vi "top level batch unzip VI.vi"() -> ()   [LabVIEW 2010]
uses:
  <vilib>/zip/NI_Unzip.lvlib
panel:
  out "UnZipping Files":bool
  out "Scanning":bool
  in  "Zip File Location":T1(ring)
  in  "save unzipped":path caption="Choose a directory to save Unzipped files into."
  in  "Unzipp":bool
  in  "Scan button":bool
  out "Number of Zip files found":i32
  in  "scan dir":path caption="Top Level to scan for *.zip files (will scan all sub directories as well)"
  in  "stop":bool
  # "BATCH UNZIP"
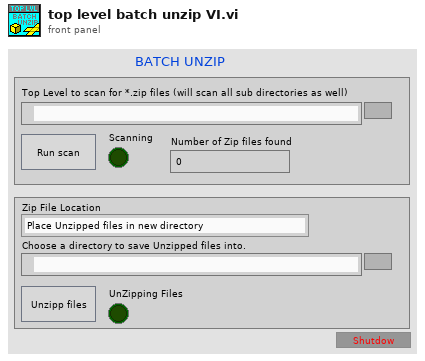
[diagram p1: front panel]
types:
  T1 = enum16{"Place Unzipped files in new directory", "Place Unzipped files in same directory as zip file"}
  T2 = enum8{"Enabled", "Disabled", "Disabled and Grayed Out"}
  T3 = enum32{"invalid app kind", "Development System", "Run Time System", "Student Edition", "Embedded LabVIEW", "Evaluation", "Custom"}
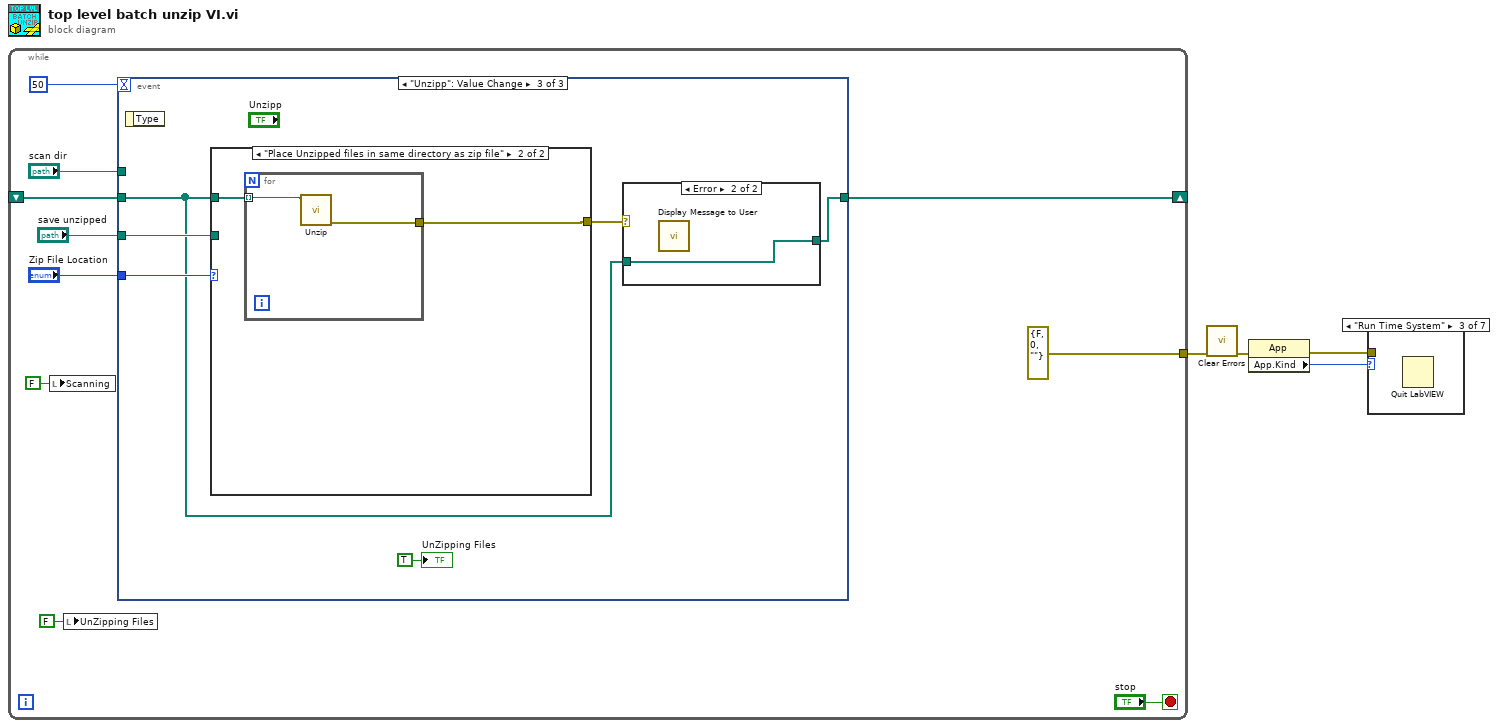
[diagram p0: block diagram]
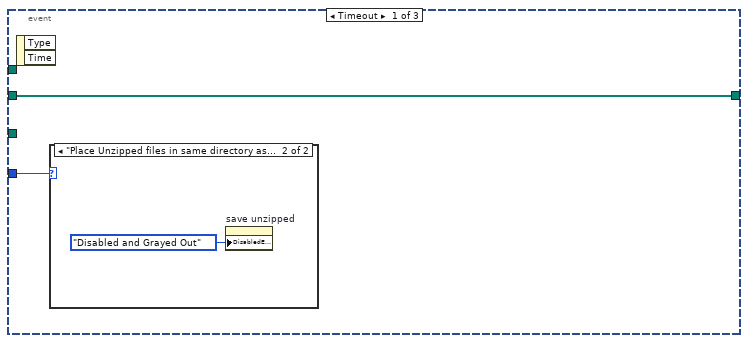
[diagram p8: hidden frame]
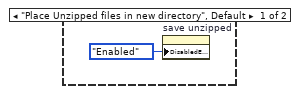
[diagram p9: hidden frame]
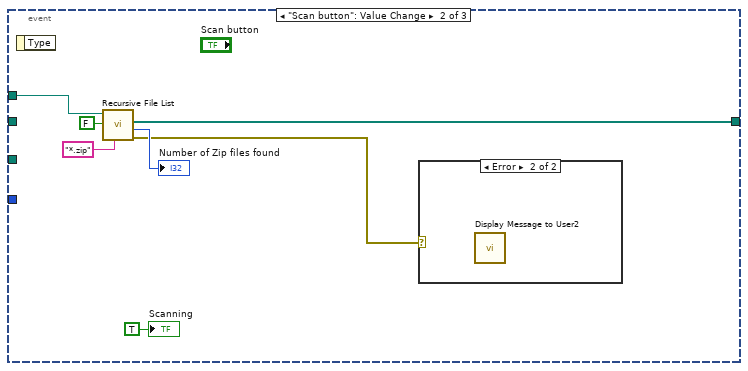
[diagram p10: hidden frame]
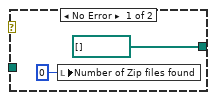
[diagram p12: hidden frame]
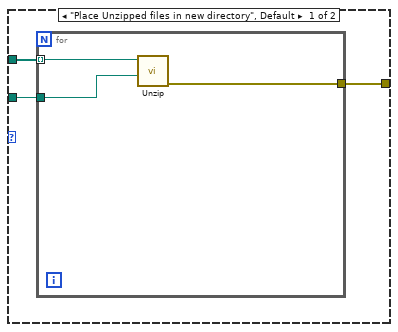
[diagram p13: hidden frame]
diagram:
  n1 = while {
    shift-right: [w12] -> _
    shift-left: _ -> [w11]
    tunnel: [errorcluster {"status"=FALSE, "code"=0, "source"=""} ("error out")] -> w1
    stop <- "stop" stop-if-true
    n2 = local write "Scanning"(FALSE ("Scanning")) -> ()
    n3 = local write "UnZipping Files"(FALSE ("UnZipping Files")) -> ()
    n4 = event shown="[2] \"Unzipp\": Value Change" {
      selector: _ -> [_ _ _]
      dyn-events: _ -> [_ _ _]
      timeout: 50 -> [_ _ _]
      tunnel: [w15 w22 w28] -> w12
      tunnel: w11 -> [w15 _ w27]
      tunnel: "scan dir" -> [_ w21 _]
      tunnel: "Zip File Location" -> [w16 _ w31]
      tunnel: "save unzipped" -> [_ _ w30]
      event Timeout {
        n5 = event-data() -> ()  [unwired: 1 in, 2 out]
        n6 = case shown="\"Place Unzipped files in same directory as zip file\"" w16 {
          frame "Place Unzipped files in new directory", Default {
            n7 = property on="save unzipped" class="Path"("DisabledEnum"=T2."Enabled" ("Disabled")) -> ()  [unwired: 2 in, 2 out]
          }
          frame "Place Unzipped files in same directory as zip file" {
            n8 = property on="save unzipped" class="Path"("DisabledEnum"=T2."Disabled and Grayed Out" ("Disabled")) -> ()  [unwired: 2 in, 2 out]
          }
        }
      }
      event "Scan button": Value Change {
        n9 = event-data() -> ()  [unwired: 1 in, 1 out]
        n10 = call <vilib>:"Recursive File List.vi"("pattern"="*.zip", "Treat LLBs as Folders?"=FALSE, "Folder Path"=w21) -> ("error out"=w20:errorcluster, "Number of Files"=→"Number of Zip files found":i32, "All Files in Dir"=w22:path[])  [unwired: 4 in, 2 out]
        n11 = case shown="Error" w20 {
          frame No Error {
          }
          frame Error {
            n12 = call "Display Message to User2"() -> ()  [unwired: 10 in, 2 out]
          }
        }
        "Scanning" <- TRUE ("Scanning")
      }
      event "Unzipp": Value Change {
        n13 = event-data() -> ()  [unwired: 1 in, 1 out]
        n14 = case shown="\"Place Unzipped files in same directory as zip file\"" w31 {
          tunnel: w27 -> [w37 w42]
          tunnel: w30 -> [w36 _]
          tunnel: [w35 w41] -> w29
          frame "Place Unzipped files in new directory", Default {
            n15 = for {
              tunnel: w37 -> [w40] mode=indexing
              tunnel: w36 -> [w39]
              tunnel: [w38] -> w35
              n16 = call <vilib>:"Unzip.vi"("Target directory (same as Zip file if empty)"=w39, "Zip file"=w40) -> ("error out"=w38:errorcluster)  [unwired: 7 in, 2 out]
            }
          }
          frame "Place Unzipped files in same directory as zip file" {
            n17 = for {
              tunnel: w42 -> [w44] mode=indexing
              tunnel: [w43] -> w41
              n18 = call <vilib>:"Unzip.vi"("Zip file"=w44) -> ("error out"=w43:errorcluster)  [unwired: 8 in, 2 out]
            }
          }
        }
        n19 = case shown="Error" w29 {
          tunnel: [path[] [] ("All Files in Dir") w34] -> w28
          tunnel: w27 -> [_ w34]
          frame No Error {
            n20 = local write "Number of Zip files found"(0 ("Number of Zip files found")) -> ()
          }
          frame Error {
            n21 = call "Display Message to User"() -> ()  [unwired: 10 in, 2 out]
          }
        }
        "UnZipping Files" <- TRUE ("UnZipping Files")
      }
    }
  }
  n22 = call <vilib>:"Clear Errors.vi"("error in (no error)"=w1) -> ("error out"=w4:errorcluster)  [unwired: 6 in]
  n23 = property class="App"(error in=w4) -> (error out=w3:errorcluster, "App.Kind"=w2:T3)  [unwired: 1 in, 1 out]
  n24 = case shown="\"Run Time System\"" w2 {
    tunnel: w3 -> [_ _ _ _ _ _ _]
    frame "invalid app kind", Default {
    }
    frame "Development System" {
    }
    frame "Run Time System" {
      n25 = Quit LabVIEW() -> ()  [unwired: 1 in]
    }
    frame "Student Edition" {
    }
    frame "Embedded LabVIEW" {
    }
    frame "Evaluation" {
    }
    frame "Custom" {
    }
  }
